vi "Compile Save Data (SubVI).vi"(0 "Dispense Mode":T5(ring), 1 "Mass Chart":T3, 2 "Relay Control":T4={"Master (All Relays)"=FALSE, "Relay1"=FALSE, "Relay2"=TRUE, "Relay3"=FALSE, "Relay4"=FALSE, "Relay5"=FALSE, "Relay6"=FALSE, "Relay7"=FALSE}, 3 "Dispense Setpoint (%)":dbl=2.5, 4 "Values":T6 {"Drain Time (s)" format="%.2f"; "Drain Rate (g/sec)" format="%.2f"; "Spray Mass Loss (g)" format="%.2f"; "Time Elapsed (s)" format="%.2f"; "Time Target (s)" format="%.2f"; "Dynamic Setpoint (g)" format="%.2f"; "Static Setpoint (g)" format="%.2f"; "Grams to Setpoint" format="%.2f"; "Adjusted Mass (g)" format="%.2f"; "Dispense Rate (g/sec)" format="%.2f"; "Fill Mass (g)" format="%.2f"; "Fill Rate (g/sec)" format="%.2f"}, 5 "Settings":T2={"ON Settings"={"Enable Dynamic Setpoint?"=TRUE, "Enable Dynamic Dispense Time?"=TRUE, "Enable Drain Rate Functions"=TRUE, "Dispense Sample Time (s)"=0.5, "Dispense Slope Ave"=0, "ON Timeout (sec)"=600.0, "1st Setpoint (% of Target)"=0.0, "2nd Setpoint (% of Target)"=0.0, "3rd Setpoint (% of Target)"=0.0, "Measure Dispense Delay (sec)"=0.0, "Settle Slope Sample Time (s)"=0.0}, "OFF Settings"={"Drain Sample Time (s)"=0.5, "Drain Rate Ave Size"=5, "Drain Rate Limits (± g/sec)"=10.0, "Level Slope Range (± g/sec)"=0.25, "OFF Timeout (sec)"=0.0, "Near SP Slope Level (± g/sec)"=0.01, "Near Setpoint Threshold (%)"=95.0}, "Overshoot Settings"={"Time Limit (s)"=60.0, "Container MAX (g)"=1500.0, "Max FILL Slope (+/- g/sec)"=10.0, "% Overshot to Enable (>)"=0.25}, "FILL Timeout (s)"=300.0, "Full Settle Time (s)"=3.0, "Pre-Hydrate \nSpray Time (s)"=10.0, "Pre-Hydrate \nWait Time (s)"=30.0}, 7 "Hydration (g)":dbl, 9 "Product Mass (g)":dbl, 11 "Product Values":T1) -> (14 "Data Array Output":dbl[](array[numeric]), 15 "Column Header Text Array":string[](array[string])=["Grams (SCB)", "Fill Target", "Dispense Target", "Relay (All)", "Relay1 (Spray)", "Relay2 (Fill)", "Relay3 (Drain)", "Relay4", "Relay5", "Relay6", "Relay7", "Dispense Mode", "Dispense Setpoint (%)", "Spray Timeout (s)", "Wait Timeout (s)", "Adjusted Mass (grams)", "Time Target (s)", "Dispense Rate (g/sec)", "Dynamic Setpoint (g)", "Measure Dispense Delay (s)", "Fill Mass (grams)", "Fill Rate (g/sec)", "Time Elapsed (s)", "Spray Mass Loss (g)"])   [LabVIEW 2012]
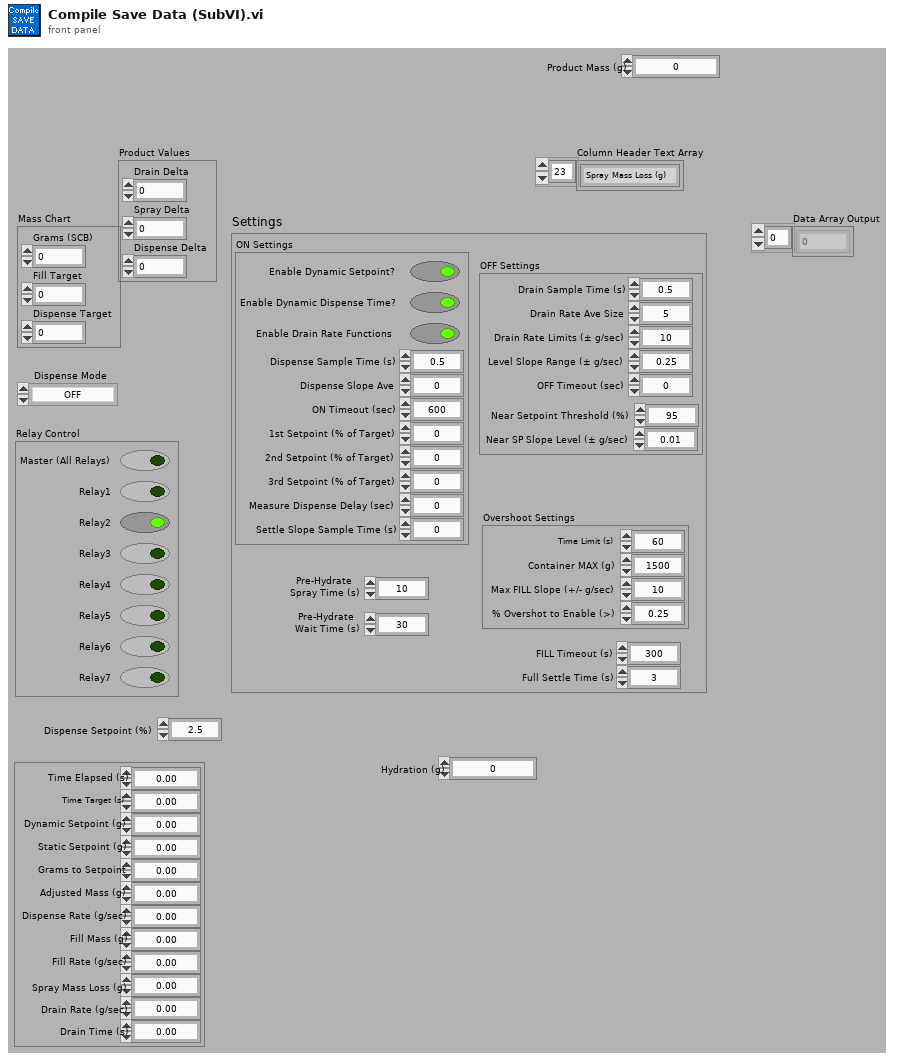
[diagram p1: front panel]
types:
  T1 = cluster{"Drain Delta":dbl, "Spray Delta":dbl, "Dispense Delta":dbl}
  T2 = cluster{"ON Settings":cluster{"Enable Dynamic Setpoint?":bool, "Enable Dynamic Dispense Time?":bool, "Enable Drain Rate Functions":bool, "Dispense Sample Time (s)":dbl, "Dispense Slope Ave":i32, "ON Timeout (sec)":dbl, "1st Setpoint (% of Target)":dbl, "2nd Setpoint (% of Target)":dbl, "3rd Setpoint (% of Target)":dbl, "Measure Dispense Delay (sec)":dbl, "Settle Slope Sample Time (s)":dbl}, "OFF Settings":cluster{"Drain Sample Time (s)":dbl, "Drain Rate Ave Size":i32, "Drain Rate Limits (± g/sec)":dbl, "Level Slope Range (± g/sec)":dbl, "OFF Timeout (sec)":dbl, "Near SP Slope Level (± g/sec)":dbl, "Near Setpoint Threshold (%)":dbl}, "Overshoot Settings":cluster{"Time Limit (s)":dbl, "Container MAX (g)":dbl, "Max FILL Slope (+/- g/sec)":dbl, "% Overshot to Enable (>)":dbl}, "FILL Timeout (s)":dbl, "Full Settle Time (s)":dbl, "Pre-Hydrate \nSpray Time (s)":dbl, "Pre-Hydrate \nWait Time (s)":dbl}
  T3 = cluster{"Grams (SCB)":dbl, "Fill Target":dbl, "Dispense Target":dbl}
  T4 = cluster{"Master (All Relays)":bool, "Relay1":bool, "Relay2":bool, "Relay3":bool, "Relay4":bool, "Relay5":bool, "Relay6":bool, "Relay7":bool}
  T5 = enum16{"OFF", "INITIAL", "FILL", "DISPENSE", "ADJUST"}
  T6 = cluster{"Time Elapsed (s)":dbl, "Time Target (s)":dbl, "Dynamic Setpoint (g)":dbl, "Static Setpoint (g)":dbl, "Grams to Setpoint":dbl, "Adjusted Mass (g)":dbl, "Dispense Rate (g/sec)":dbl, "Fill Mass (g)":dbl, "Fill Rate (g/sec)":dbl, "Spray Mass Loss (g)":dbl, "Drain Rate (g/sec)":dbl, "Drain Time (s)":dbl}
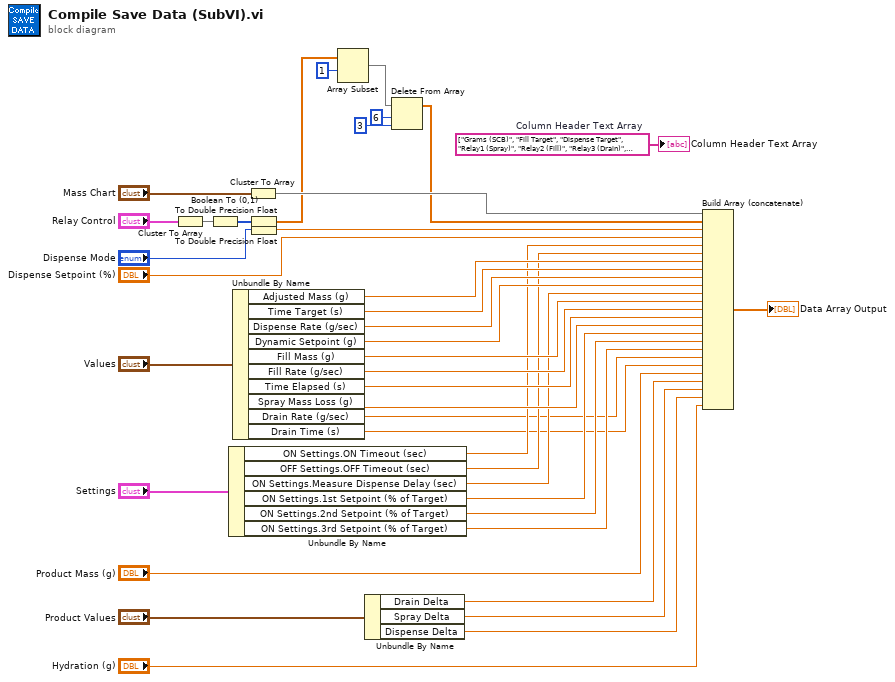
[diagram p0: block diagram]
diagram:
  w18 = string[] ["Grams (SCB)", "Fill Target", "Dispense Target", "Relay1 (Spray)", "Relay2 (Fill)", "Relay3 (Drain)", "Dispense Mode", "Dispense Setpoint (%)", "Spray Timeout (s)", "Wait Timeout (s)", "Adjusted Mass (grams)", "Time Target (s)", "Dispense Rate (g/sec)", "Dynamic Setpoint (g)", "Measure Dispense Delay (s)", "Fill Mass (grams)", "Fill Rate (g/sec)", "Time Elapsed (s)", "Spray Mass Loss (g)", "SP 1 (%)", "SP2 (%)", "SP3 (%)", "Drain Rate (g/sec)", "Drain Time (s)", "Product Mass (g)", "Drain Delta (g)", "Spray Delta (g)", "Dispense Delta (g)", "Hydration (g)"]  # Column Header Text Array
  n1 = Cluster To Array(cluster="Relay Control") -> (array=w19:bool[])
  n2 = Boolean To (0,1)(Boolean=w19) -> (0, 1=w20:i16[])
  n3 = Unbundle By Name("Settings") -> ("ON Settings.ON Timeout (sec)"=w24:dbl, "OFF Settings.OFF Timeout (sec)"=w25:dbl, "ON Settings.Measure Dispense Delay (sec)"=w26:dbl, "ON Settings.1st Setpoint (% of Target)"=w17:dbl, "ON Settings.2nd Setpoint (% of Target)"=w16:dbl, "ON Settings.3rd Setpoint (% of Target)"=w15:dbl)
  n4 = Unbundle By Name("Values") -> ("Adjusted Mass (g)"=w27:dbl, "Time Target (s)"=w28:dbl, "Dispense Rate (g/sec)"=w29:dbl, "Dynamic Setpoint (g)"=w30:dbl, "Fill Mass (g)"=w31:dbl, "Fill Rate (g/sec)"=w32:dbl, "Time Elapsed (s)"=w33:dbl, "Spray Mass Loss (g)"=w34:dbl, "Drain Rate (g/sec)"=w14:dbl, "Drain Time (s)"=w13:dbl)
  n5 = Cluster To Array(cluster="Mass Chart") -> (array=w21:dbl[])
  n6 = To Double Precision Float(number=w20) -> (double precision float=w10:dbl[])
  n7 = To Double Precision Float(number="Dispense Mode") -> (double precision float=w23:dbl)
  n8 = Array Subset(array=w10, index=1) -> (w8:dbl[])  [unwired: 1 in]
  n9 = Unbundle By Name("Product Values") -> ("Drain Delta"=w4:dbl, "Spray Delta"=w3:dbl, "Dispense Delta"=w2:dbl)
  n10 = Delete From Array(array=w8, length=6, index=3) -> (array with subset deleted=w7:dbl[])  [unwired: 1 out]
  n11 = Build Array (concatenate)(w21, w7, w23, "Dispense Setpoint (%)", w24, w25, w27, w28, w29, w30, w26, w31, w32, w33, w34, w17, w16, w15, w14, w13, "Product Mass (g)", w4, w3, w2, "Hydration (g)") -> (→"Data Array Output":dbl[])
  "Column Header Text Array" <- w18
